vi "SelectPrinter.vi"() -> (0 "ChosenPrinter":string, 1 "Closed?":bool=TRUE)   [LabVIEW 2018]
uses:
  Type/_RT Command.ctl
  <vilib>/Utility/NIReport.llb/NI_ReportGenerationCore.lvlib
panel:
  in  "OK":bool
  in  "Printers":u16(ring)=1 items=["Send To OneNote 2016", "OneNote", "Microsoft XPS Document Writer", "Microsoft Print to PDF", "Fax", "\\\\woop01\\Xerox 9302 Global Print Driver PCL6"]
  # "Please select a printer from the drop-down list below and click OK"
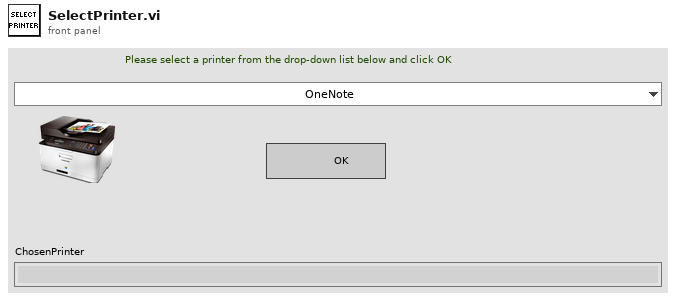
[diagram p1: front panel]
types:
  T1 = typedef "_RT Command.ctl" = enum16{"xml Start Run", "xml Start Actual Run", "xml Stop Run", "xml Runtime Update", "xml Get Status", "xml Get Table", "xml Set Table", "xml Get Configuration", "xml System Status", "xml Set LC Input Logic", "xml Get Data", "xml Get Info", "Start", "StartActualRun", "Stop", "Runtime Update", "Get Data", "Get Info", "Get Status", "Get Param", "Get Config", "Get Table", "Read ADC", "Set Oscillator", "Update Config", "Update Table", "Set All Pol", "Set Pol and DC", "Set Max Mass", "Toggle RP", "Toggle EL", "Set PIC", "Initialize Turbo", "Send Turbo Comm", "Close Turbo", "P1", "P2", "P3", "Send Serial", "Set LC Out", "Get LC In", "Read VAC", "Test Table", "Toggle Power", "Get Startup", "Set Startup", "Get ADC Table", "Set ADC Table", "Get Brief Status", "Get Detail Status", "Auxiliary Update", "Set CC Logics", "Set CC Input Logics", "Ignore Error", "invalid"}
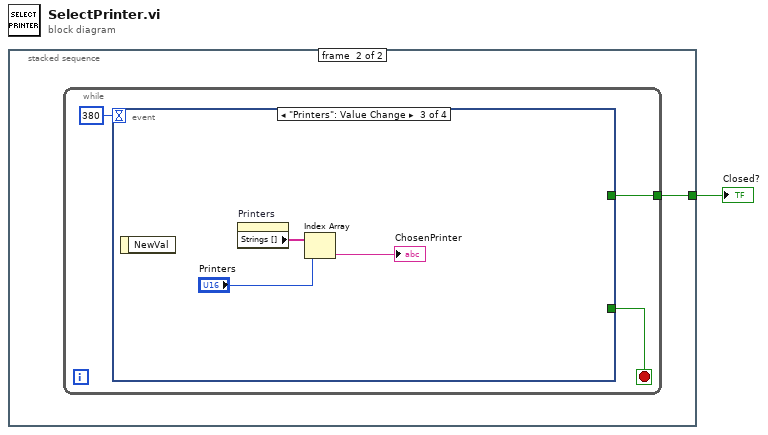
[diagram p0: block diagram]
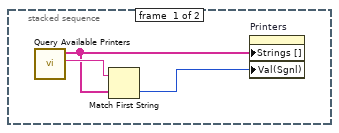
[diagram p2: hidden frame]
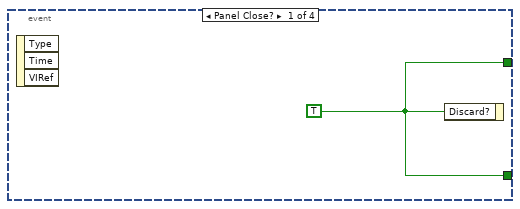
[diagram p3: hidden frame]
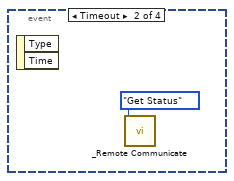
[diagram p4: hidden frame]
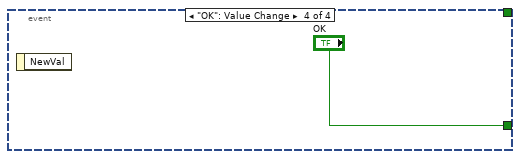
[diagram p5: hidden frame]
diagram:
  n1 = stacked-sequence {
    tunnel: [_ w5] -> w1
    frame #0 {
      n2 = call <vilib>:"Query Available Printers.vi"() -> ("default printer"=w4:string, "system configured printers"=w3:string[])  [unwired: 9 in, 1 out]
      n3 = Match First String(2:w3, 3:w4) -> (0:w2:i32)  [unwired: 1 out]
      n4 = property on="Printers" class="Ring (strict)"("Strings []"=w3, "Val(Sgnl)"=w2) -> ()  [unwired: 2 in, 2 out]
    }
    frame #1 {
      n5 = while {
        tunnel: [w6] -> w5
        stop <- w8 stop-if-true
        n6 = event shown="[2] \"Printers\": Value Change" {
          selector: _ -> [_ _ _ _]
          dyn-events: _ -> [_ _ _ _]
          timeout: 380 -> [_ _ _ _]
          tunnel: [w9 _ _ "OK"] -> w8
          tunnel: [w9 _ _ _] -> w6
          event Panel Close? {
            w9 = TRUE
            n7 = event-data() -> ()  [unwired: 1 in, 3 out]
            n8 = event-data("Discard?"=w9) -> ()  [unwired: 1 in, 1 out]
          }
          event Timeout {
            n9 = event-data() -> ()  [unwired: 1 in, 2 out]
            n10 = call "_Remote Communicate.vi"("Command"=_RT_Command."Get Status") -> ()  [unwired: 5 in, 4 out]
          }
          event "Printers": Value Change {
            n11 = event-data() -> ()  [unwired: 1 in, 1 out]
            n12 = property on="Printers" class="Ring (strict)"() -> ("Strings []"=w13:string[])  [unwired: 2 in, 2 out]
            n13 = Index Array(array=w13, index="Printers") -> (element=→"ChosenPrinter":string)
          }
          event "OK": Value Change {
            n14 = event-data() -> ()  [unwired: 1 in, 1 out]
          }
        }
      }
    }
  }
  "Closed?" <- w1
